vi "HoppingStep(XYWithin_And_Nonlinear).vi"() -> ()   [LabVIEW 2014]
uses:
  <vilib>/Platform/TimedLoop/XDataNode/timing_clust.ctl
  <vilib>/Platform/TimedLoop/XDataNode/nitl_modes.ctl
  <vilib>/Platform/TimedLoop/XDataNode/wakeup.ctl
  <vilib>/rvi/Emulation/niFpgaGetClockAttributes.vi
  <vilib>/rvi/Emulation/niFpgaSctlEmulationGetInTimedLoop.vi
  <vilib>/rvi/Emulation/niFpgaEmulationReportErrorSimple.vi
  <vilib>/rvi/eio/common/nirviEmuTemplateMethod_errors.vi
  <vilib>/rvi/Emulation/niFpgaProcessEmulError.vi
  <vilib>/rvi/Emulation/niFpgaCriticalErrorInLSC.vi
  <vilib>/rvi/interface/RandomDataEmulation/niFpgaRandomDataHandleErrors.vi
  <vilib>/eio/EIONode/EIONode.xnode
  <vilib>/Platform/TimedLoop/XDataNode/XDataNode.xnode
  <vilib>/rvi/DataTransferAndStorage/Container/XNode/niFpgaContainer.xnode
  <vilib>/rvi/interface/RandomDataEmulation/nirviRandomDataFpgaReadWriteTemplate.vi
  <vilib>/Platform/TimedLoop/XDataNode/XDNodeRunTimeDep.lvlib
panel:
  out "Z":i32
  in  "MajorWithdraw":i16
  in  "ZOffset":i16
  in  "stop":bool
  out "PresZDia":i32(graph)
  in  "XNum":i16
  in  "XStepIndex":i16
  in  "XOffset":i16
  in  "YNum":i16
  in  "YStepIndex":i16
  in  "YOffset":i16
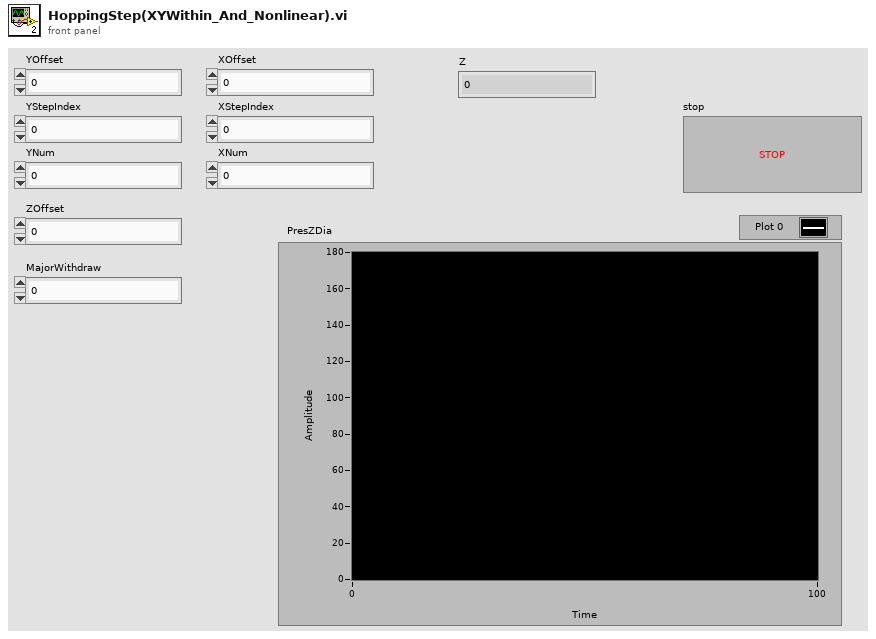
[diagram p1: front panel]
types:
  T1 = typedef "XDNodeRunTimeDep.lvlib/timing_clust.ctl" = cluster{"Expected End [f-1]":u64, "Actual End [f-1]":u64, "Finished Late? [f-1]":bool, "Expected End [i-1]":u64, "Actual End [i-1]":u64, "Finished Late? [i-1]":bool, "Expected Start [i]":u64, "Actual Start [i]":u64, "Expected Start [f]":u64, "Actual Start [f]":u64, "Source Name":string, "Structure Name":string, "Period":i64, "Deadline":i64, "Offset":i64, "Start":i64, "Priority":i32, "Timeout":i32, "Mode":T2, "Wakeup Reason":T3, "Error":errorcluster, "Source Type":string, "Secondary Source Type":string, "Global End Time":u64, "Global Start Time":u64, "Frame Duration":u64, "Iteration Duration":u64, "Assigned CPU":i32, "I/O Scan Engine Mode":u32}
  T2 = typedef "XDNodeRunTimeDep.lvlib/nitl_modes.ctl" = enum32{"No Change", "Process missed periods, maintain original phase", "Discard missed periods, maintain original phase", "Process missed periods, ignore original phase", "Discard missed periods, ignore original phase"}
  T3 = typedef "XDNodeRunTimeDep.lvlib/wakeup.ctl" = enum32{"Normal", "Aborted", "Asynchronous wakeup", "Timing source error", "Timed loop error", "Timeout"}
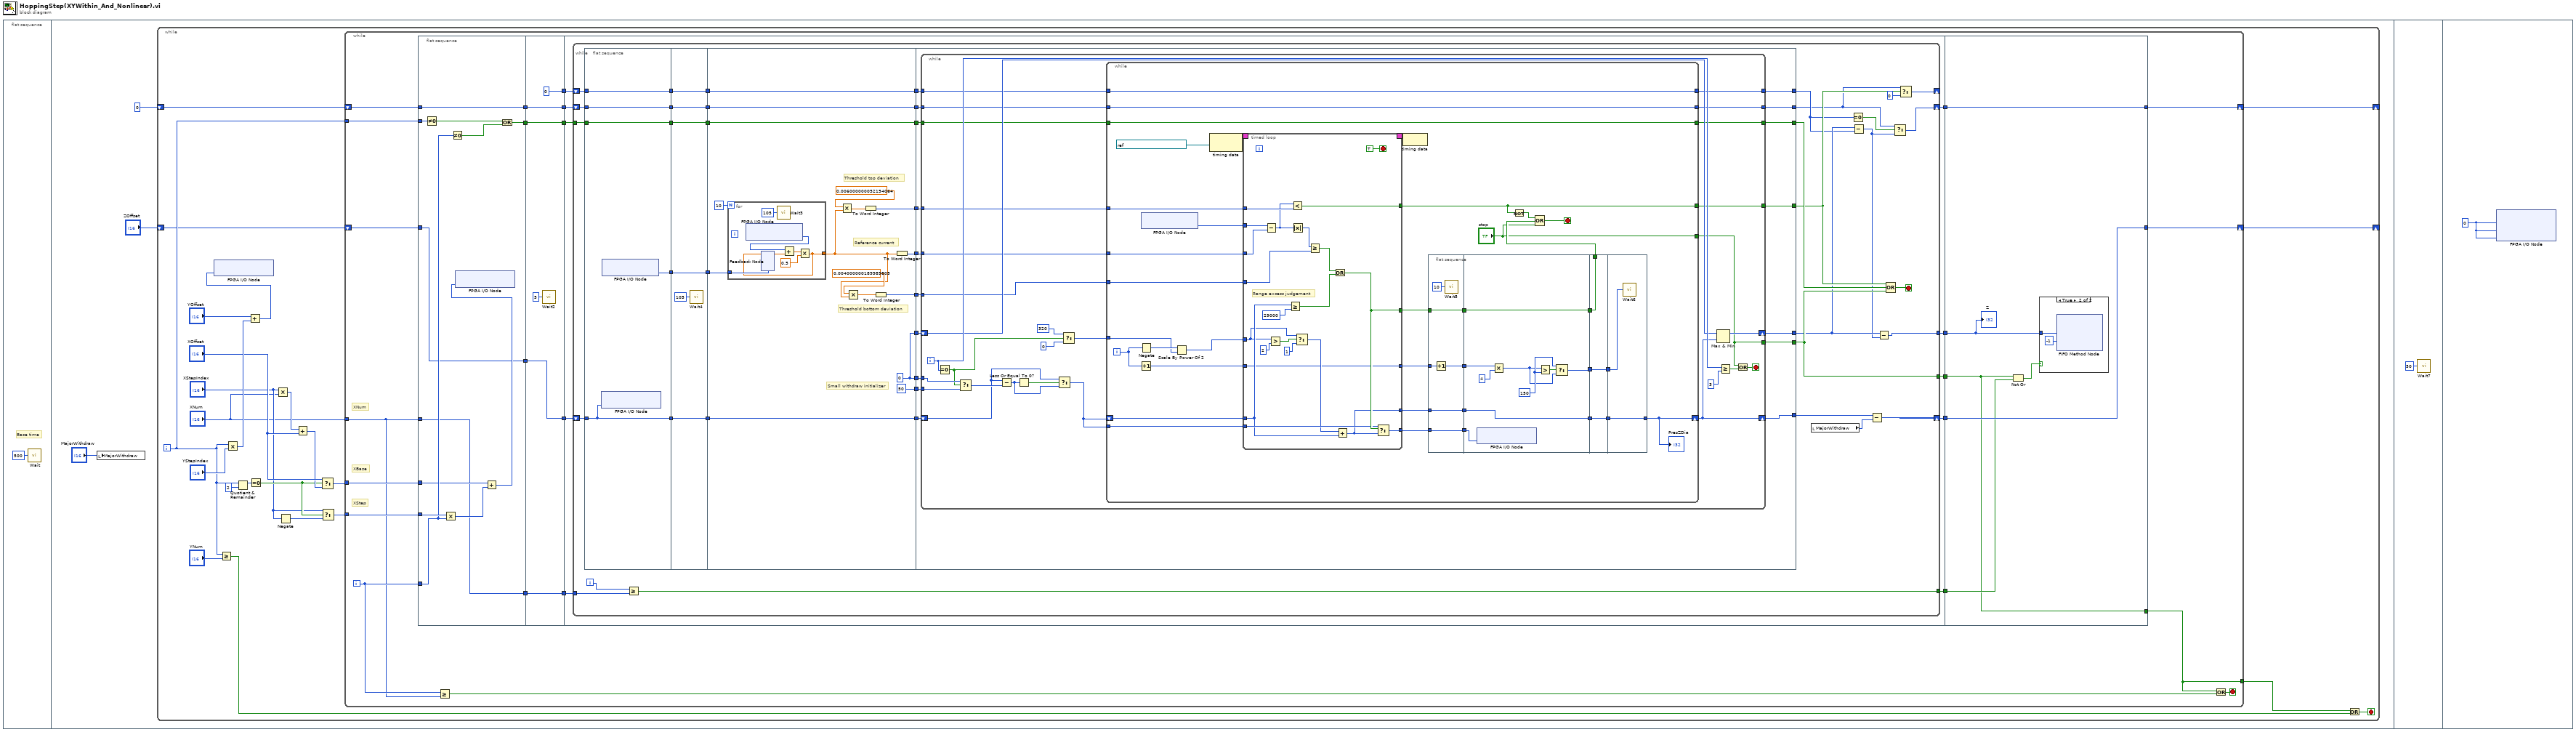
[diagram p0: block diagram]
diagram:
  n1 = flat-sequence {
    frame #0 {
      # "Base time"
      n2 = call "Wait"("Count(mSec)"=u32 500) -> ()  [unwired: 1 out]
    }
    frame #1 {
      n3 = local write "MajorWithdraw"("MajorWithdraw") -> ()
      n4 = while {
        shift-right: [w7] -> _
        shift-left: "ZOffset" -> [w9]
        shift-right: [w5] -> _
        shift-left: i16 0 -> [w8]
        i -> [w10]
        stop <- w25 stop-if-true
        n5 = Greater Or Equal?(x=w10, y="YNum") -> (x >= y?=w23:bool)
        n6 = Multiply(x=w10, y="YStepIndex") -> (x*y=w26:i32)
        n7 = Quotient & Remainder(x=w10, y=2) -> (x-y*floor(x/y)=w20:i32)  [unwired: 1 out]
        n8 = Add(x="YOffset", y=w26) -> (x+y=w22:i32)
        n9 = xnode "FPGA I/O Node"("Connector0/AO3"=w22) -> ()  [unwired: 1 in, 1 out]
        n10 = Equal To 0?(x=w20) -> (x = 0?=w15:bool)
        n11 = Multiply(x="XStepIndex", y="XNum") -> (x*y=w19:i16)
        n12 = Negate(x="XStepIndex") -> (-x=w13:i16)
        n13 = Add(x=w19, y="XOffset") -> (x+y=w17:i16)
        n14 = Select(t="XOffset", s=w15, f=w17) -> (s? t:f=w16:i16)
        n15 = Select(t="XStepIndex", s=w15, f=w13) -> (s? t:f=w12:i16)
        n16 = while {
          tunnel: w16 -> [w54]
          tunnel: w12 -> [w53]
          tunnel: "XNum" -> [w33]
          tunnel: w10 -> [w52]
          shift-right: [w44] -> w7
          shift-left: w9 -> [w49]
          shift-right: [w29] -> w5
          shift-left: w8 -> [w41]
          tunnel: [w31] -> w6
          i -> [w34]
          stop <- w35 stop-if-true
          # "XNum"
          # "XStep"
          # "XBase"
          n17 = flat-sequence {
            tunnel: w33 -> [w56]
            tunnel: w54 -> [w57]
            tunnel: w53 -> [w66]
            tunnel: w34 -> [w62]
            tunnel: w52 -> [w63]
            tunnel: [w59] -> w51
            tunnel: w49 -> [w58]
            tunnel: [w58] -> w48
            tunnel: [w56] -> w42
            tunnel: w41 -> [w55]
            tunnel: [w55] -> w39
            tunnel: w51 -> [w70]
            tunnel: [w71] -> w50
            tunnel: w48 -> [w71]
            tunnel: [w70] -> w47
            tunnel: [w69] -> w43
            tunnel: w42 -> [w69]
            tunnel: [w68] -> w40
            tunnel: w39 -> [w68]
            tunnel: [i16 0] -> w36
            tunnel: w50 -> [w82]
            tunnel: w47 -> [w81]
            tunnel: [w80] -> w46
            tunnel: [w79] -> w45
            tunnel: w43 -> [w78]
            tunnel: w40 -> [w77]
            tunnel: [w76] -> w38
            tunnel: [w75] -> w37
            tunnel: w36 -> [w74]
            tunnel: [w73] -> w30
            tunnel: w46 -> [w295]
            tunnel: w45 -> [w294]
            tunnel: [w294] -> w44
            tunnel: w38 -> [w291]
            tunnel: w37 -> [w293]
            tunnel: [w291] -> w31
            tunnel: w30 -> [w290]
            tunnel: [w290] -> w29
            frame #0 {
              n18 = Not Equal To 0?(x=w63) -> (x != 0?=w61:bool)
              n19 = Multiply(x=w66, y=w62) -> (x*y=w65:i32)
              n20 = Not Equal To 0?(x=w62) -> (x != 0?=w60:bool)
              n21 = Add(x=w57, y=w65) -> (x+y=w64:i32)
              n22 = xnode "FPGA I/O Node"("Connector0/AO2"=w64) -> ()  [unwired: 1 in, 1 out]
              n23 = Or(x=w61, y=w60) -> (x .or. y?=w59:bool)
            }
            frame #1 {
              n24 = call "Wait2"("Count(uSec)"=u32 5) -> ()  [unwired: 1 out]
            }
            frame #2 {
              n25 = while {
                shift-right: [w112] -> w79
                shift-left: w82 -> [w115]
                tunnel: [w96] -> w80
                tunnel: w81 -> [w111]
                tunnel: [w107] -> w76
                tunnel: w78 -> [w105]
                shift-right: [w87] -> w73
                shift-left: w77 -> [w103]
                tunnel: [w99] -> w75
                shift-right: [w91] -> _
                shift-left: w74 -> [w95]
                i -> [w104]
                stop <- w106 stop-if-true
                n26 = flat-sequence {
                  tunnel: [w130] -> w124
                  tunnel: [w129] -> w116
                  tunnel: w115 -> [w129]
                  tunnel: w111 -> [w128]
                  tunnel: [w128] -> w109
                  tunnel: w103 -> [w127]
                  tunnel: [w127] -> w101
                  tunnel: w95 -> [w126]
                  tunnel: [w126] -> w94
                  tunnel: [w136] -> w125
                  tunnel: w124 -> [w136]
                  tunnel: [w134] -> w117
                  tunnel: w116 -> [w134]
                  tunnel: [w133] -> w110
                  tunnel: w109 -> [w133]
                  tunnel: [w132] -> w102
                  tunnel: w101 -> [w132]
                  tunnel: w94 -> [w131]
                  tunnel: [w131] -> w93
                  tunnel: w125 -> [w151]
                  tunnel: [w148] -> w123
                  tunnel: [w147] -> w122
                  tunnel: [w143] -> w121
                  tunnel: [w141] -> w120
                  tunnel: [i16 50] -> w119
                  tunnel: [w141] -> w118
                  tunnel: w117 -> [w140]
                  tunnel: [w140] -> w114
                  tunnel: w110 -> [w139]
                  tunnel: [w139] -> w108
                  tunnel: w102 -> [w138]
                  tunnel: [w138] -> w100
                  tunnel: w93 -> [w137]
                  tunnel: [w137] -> w92
                  tunnel: w123 -> [w173]
                  tunnel: w122 -> [w174]
                  tunnel: w121 -> [w165]
                  tunnel: w120 -> [w176]
                  tunnel: w119 -> [w175]
                  tunnel: w118 -> [w172]
                  tunnel: w114 -> [w171]
                  tunnel: [w170] -> w113
                  tunnel: [w169] -> w88
                  tunnel: w108 -> [w168]
                  tunnel: [w167] -> w97
                  tunnel: [w166] -> w107
                  tunnel: [w164] -> w90
                  tunnel: w100 -> [w163]
                  tunnel: [w162] -> w84
                  tunnel: w92 -> [w161]
                  tunnel: [w160] -> w86
                  frame #0 {
                    n27 = xnode "FPGA I/O Node"("Connector0/AO0"=w129) -> ()  [unwired: 1 in, 1 out]
                    n28 = xnode "FPGA I/O Node"() -> ("Connector0/AI1"=w130:i16)  [unwired: 1 in, 1 out]
                  }
                  frame #1 {
                    n29 = call "Wait4"("Count(uSec)"=u32 105) -> ()  [unwired: 1 out]
                  }
                  frame #2 {
                    w141 = i16 0
                    # "Small withdraw initializer"
                    # "Threshold top deviation"
                    # "Threshold bottom deviation"
                    # "Reference current"
                    n30 = for {
                      N: 10 -> [_]
                      tunnel: w151 -> [w158]
                      tunnel: [w153] -> w145
                      n31 = xnode "FPGA I/O Node"() -> ("Connector0/AI1"=w156:i16)  [unwired: 1 in, 1 out]
                      n32 = feedback #1(w158) -> (w157:sgl)
                      n33 = call "Wait3"("Count(uSec)"=u32 105) -> ()  [unwired: 1 out]
                      n34 = Add(x=w156, y=w157) -> (x+y=w155:sgl)
                      n35 = Multiply(x=w155, y=sgl 0.5) -> (x*y=w153:sgl)
                      n36 = feedback-in #1(w153) -> ()
                    }
                    n37 = Multiply(x=sgl 0.006, y=w145) -> (x*y=w144:sgl)
                    n38 = Multiply(x=sgl 0.004, y=w145) -> (x*y=w149:sgl)
                    n39 = To Word Integer(number=w144) -> (16bit integer=w143:i16)
                    n40 = To Word Integer(number=w149) -> (16bit integer=w148:i16)
                    n41 = To Word Integer(number=w145) -> (16bit integer=w147:i16)
                  }
                  frame #3 {
                    n42 = while {
                      tunnel: [w177] -> w166
                      shift-right: [w195] -> w170
                      shift-left: w171 -> [w199]
                      tunnel: w176 -> [w197]
                      shift-right: [w194] -> w169
                      shift-left: w172 -> [w196]
                      tunnel: w175 -> [w189]
                      tunnel: w174 -> [w188]
                      tunnel: w173 -> [w187]
                      tunnel: w168 -> [w186]
                      tunnel: [w185] -> w167
                      tunnel: w165 -> [w184]
                      tunnel: [w183] -> w164
                      tunnel: w163 -> [w182]
                      tunnel: [w181] -> w162
                      tunnel: w161 -> [w180]
                      tunnel: [w179] -> w160
                      i -> [w202]
                      stop <- w204 stop-if-true
                      n43 = Equal To 0?(x=w202) -> (x = 0?=w193:bool)
                      n44 = Select(t=w197, s=w193, f=w189) -> (s? t:f=w201:i16)
                      n45 = Subtract(x=w199, y=w201) -> (x-y=w198:i32)
                      n46 = Less Or Equal To 0?(x=w198) -> (x <= 0?=w200:bool)
                      n47 = Select(t=w199, s=w200, f=w198) -> (s? t:f=w178:i32)
                      n48 = Select(t=i16 320, s=w193, f=i16 0) -> (s? t:f=w190:i16)
                      n49 = while {
                        tunnel: ["stop"] -> w177
                        shift-right: [w229] -> w195
                        shift-left: w178 -> [w235]
                        tunnel: w178 -> [w232]
                        tunnel: w190 -> [w219]
                        tunnel: w188 -> [w216]
                        tunnel: w187 -> [w215]
                        tunnel: w186 -> [w214]
                        tunnel: [w214] -> w185
                        tunnel: w184 -> [w213]
                        tunnel: [w210] -> w183
                        tunnel: w182 -> [w206]
                        tunnel: [w206] -> w181
                        tunnel: w180 -> [w207]
                        tunnel: [w207] -> w179
                        i -> [w217]
                        stop <- w208 stop-if-true
                        n50 = Increment(x=w217) -> (x+1=w221:i32)
                        n51 = Negate(x=w217) -> (-x=w220:i32)
                        n52 = xnode "FPGA I/O Node"() -> ("Connector0/AI1"=w238:i16)  [unwired: 1 in, 1 out]
                        n53 = Scale By Power Of 2(n=w220, x=w219) -> (x*2^n=w218:i16)
                        n54 = node-c288(refnum<k21> "40 MHz Onboard Clock" ("Source Name")) -> (w241:T1)
                        n55 = timed-loop {
                          timing: w241 -> [_]
                          timing-out: [_] -> w240
                          tunnel: w215 -> [w281]
                          tunnel: w238 -> [w265]
                          tunnel: [w278] -> w236
                          tunnel: [w277] -> w234
                          tunnel: w235 -> [w274]
                          tunnel: w232 -> [w276]
                          tunnel: [w273] -> w231
                          tunnel: w218 -> [w268]
                          tunnel: [w270] -> w222
                          tunnel: w221 -> [w270]
                          tunnel: w216 -> [w266]
                          tunnel: w213 -> [w264]
                          tunnel: [w262] -> w210
                          stop <- TRUE stop-if-true
                          # "Range excess judgement"
                          n56 = Subtract(x=w265, y=w266) -> (x-y=w263:i16)
                          n57 = Greater?(x=w268, y=i16 2) -> (0:w267:bool)
                          n58 = Greater Or Equal?(x=w274, y=i16 29000) -> (x >= y?=w279:bool)
                          n59 = Less?(x=w263, y=w264) -> (x < y?=w262:bool)
                          n60 = Absolute Value(x=w263) -> (abs(x)=w282:i16)
                          n61 = Select(t=w268, s=w267, f=1) -> (s? t:f=w271:i32)
                          n62 = Greater Or Equal?(x=w282, y=w281) -> (x >= y?=w280:bool)
                          n63 = Or(x=w280, y=w279) -> (x .or. y?=w277:bool)
                          n64 = Add(x=w271, y=w274) -> (x+y=w273:i32)
                          n65 = Select(t=w276, s=w277, f=w273) -> (s? t:f=w278:i32)
                        }
                        n66 = node-c288(w240) -> ()
                        n67 = flat-sequence {
                          tunnel: [w246] -> w237
                          tunnel: w236 -> [w246]
                          tunnel: w234 -> [w245]
                          tunnel: [w245] -> w233
                          tunnel: w231 -> [w244]
                          tunnel: [w244] -> w230
                          tunnel: [w243] -> w223
                          tunnel: w222 -> [w242]
                          tunnel: w237 -> [w252]
                          tunnel: [w256] -> w228
                          tunnel: w233 -> [w255]
                          tunnel: w230 -> [w256]
                          tunnel: [w255] -> w226
                          tunnel: [w248] -> w224
                          tunnel: w223 -> [w253]
                          tunnel: w228 -> [w259]
                          tunnel: [w259] -> w227
                          tunnel: w226 -> [w258]
                          tunnel: [w258] -> w212
                          tunnel: [w257] -> w225
                          tunnel: w224 -> [w257]
                          tunnel: w227 -> [w261]
                          tunnel: [w261] -> w229
                          tunnel: w225 -> [w260]
                          frame #0 {
                            n68 = Increment(x=w242) -> (x+1=w243:i32)
                            n69 = call "Wait5"("Count(uSec)"=u32 10) -> ()  [unwired: 1 out]
                          }
                          frame #1 {
                            w250 = i16 150
                            n70 = xnode "FPGA I/O Node"("Connector0/AO0"=w252) -> ()  [unwired: 1 in, 1 out]
                            n71 = Multiply(x=w253, y=i16 4) -> (x*y=w249:i32)
                            n72 = Greater?(x=w249, y=w250) -> (0:w251:bool)
                            n73 = Select(t=w250, s=w251, f=w249) -> (s? t:f=w248:i32)
                          }
                          frame #2 {
                          }
                          frame #3 {
                            n74 = call "Wait6"("Count(uSec)"=w260) -> ()  [unwired: 1 out]
                          }
                        }
                        n75 = Not(x=w210) -> (.not. x?=w209:bool)
                        n76 = Compound Arithmetic op=OR(w209, w212, "stop") -> (w208:bool)
                        "PresZDia" <- w229
                      }
                      n77 = Max & Min(x=w196, y=w195) -> (max(x,y)=w194:i32)  [unwired: 1 out]
                      n78 = Greater Or Equal?(x=w202, y=3) -> (x >= y?=w203:bool)
                      n79 = Or(x=w177, y=w203) -> (x .or. y?=w204:bool)
                    }
                  }
                }
                n80 = Greater Or Equal?(x=w104, y=w105) -> (x >= y?=w99:bool)
                n81 = local read "MajorWithdraw"() -> (w98:i16)
                n82 = Equal To 0?(x=w86) -> (x = 0?=w85:bool)
                n83 = Subtract(x=w88, y=w86) -> (x-y=w83:i32)
                n84 = Subtract(x=w113, y=w98) -> (x-y=w112:i32)
                n85 = Subtract(x=w88, y=w83) -> (x-y=w96:i32)
                n86 = Compound Arithmetic op=OR(w90, w97, w107) -> (w106:bool)
                n87 = Select(t=w84, s=w85, f=w83) -> (s? t:f=w87:i32)
                n88 = Select(t=w84, s=w90, f=i16 0) -> (s? t:f=w91:i32)
              }
            }
            frame #3 {
              n89 = Not Or(1:w293, 2:w291) -> (0:w292:bool)
              n90 = case shown="True" w292 {
                tunnel: w295 -> [_ w297]
                frame False {
                }
                frame True {
                  n91 = xnode ("FIFO Method Node")("Element"=w297, "Timeout"=-1) -> ()  [unwired: 1 in, 2 out]
                }
              }
              "Z" <- w295
            }
          }
          n92 = Greater Or Equal?(x=w34, y=w33) -> (x >= y?=w32:bool)
          n93 = Or(x=w31, y=w32) -> (x .or. y?=w35:bool)
        }
        n94 = Or(x=w6, y=w23) -> (x .or. y?=w25:bool)
      }
    }
    frame #2 {
      n95 = call "Wait7"("Count(uSec)"=u32 50) -> ()  [unwired: 1 out]
    }
    frame #3 {
      w299 = i16 0
      n96 = xnode "FPGA I/O Node"("Connector0/AO0"=w299, "Connector0/AO2"=w299, "Connector0/AO3"=w299) -> ()  [unwired: 3 in, 3 out]
    }
  }
